vi "Configure Arbitrary Sequence [SEQ] Core.vi"(5 "offset (0.00 V)":dbl[unit] format="%.4f", 7 "gain (1.00)":dbl=1.0 format="%.4f", 8 "error in (no error)":errorcluster, 9 "sequence handle (0)":i32, 10 "channel name (\"CHANNEL1\")":string="CHANNEL1", 11 "CS++Fgen in":refnum<class "CS++Fgen.lvclass">) -> (0 "error out":errorcluster, 3 "CS++Fgen out":refnum<class "CS++Fgen.lvclass">)   [LabVIEW 2013, in "CS++Fgen.lvlib" / "CS++Fgen.lvclass"]
doc: "This VI configures the properties of the function generator that affect arbitrary sequence generation. These properties are the arbitrary sequence handle, gain, and offset.\n\nNotes:\n\n(1) This VI is part of the IviFgenArbSeq [SEQ] extension group."
uses:
  CS++Fgen.lvclass
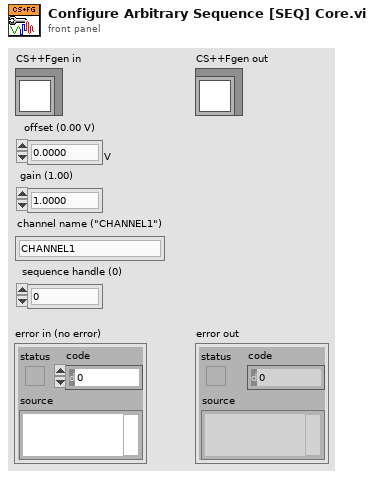
[diagram p1: front panel]
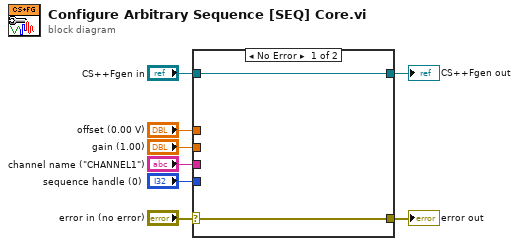
[diagram p0: block diagram]
diagram:
  n1 = case shown="No Error" "error in (no error)" {
    selector: "error in (no error)" -> [w9 w12]
    tunnel: [w9 w12] -> w7
    tunnel: [w10 w11] -> w5
    tunnel: "CS++Fgen in" -> [w10 w11]
    tunnel: "channel name (\"CHANNEL1\")" -> [_ _]
    tunnel: "offset (0.00 V)" -> [_ _]
    tunnel: "gain (1.00)" -> [_ _]
    tunnel: "sequence handle (0)" -> [_ _]
    frame No Error {
    }
    frame Error {
    }
  }
  "error out" <- w7
  "CS++Fgen out" <- w5
